vi "Create.vi"(8 "error in (no error)":errorcluster, 10 "Channel":T1=1 items=["ENC1"=1, "ENC2"=2], 11 "connection ID":i32=-1) -> (0 "error out":errorcluster, 3 "Task out":refnum<class "Encoder.lvclass">)   [LabVIEW 2009, in "MicroDAQ.lvlib" / "Encoder.lvclass"]
uses:
  <instrlib>/MicroDAQ/Channel/Encoder/Encoder.lvclass
  <instrlib>/MicroDAQ/Tools/Encoder type.ctl
  <instrlib>/MicroDAQ/Channel/Encoder/Encoder.lvclass/Encoder.ctl
  <instrlib>/MicroDAQ/Mlink library wraper/mlink.lvlib
  <instrlib>/MicroDAQ/Channel/Channel.lvclass
  <instrlib>/MicroDAQ/MicroDAQ.lvlib
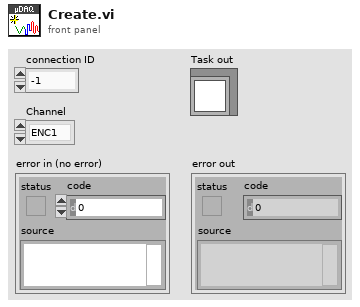
[diagram p1: front panel]
types:
  T1 = typedef "MicroDAQ.lvlib/Encoder type.ctl" = u8
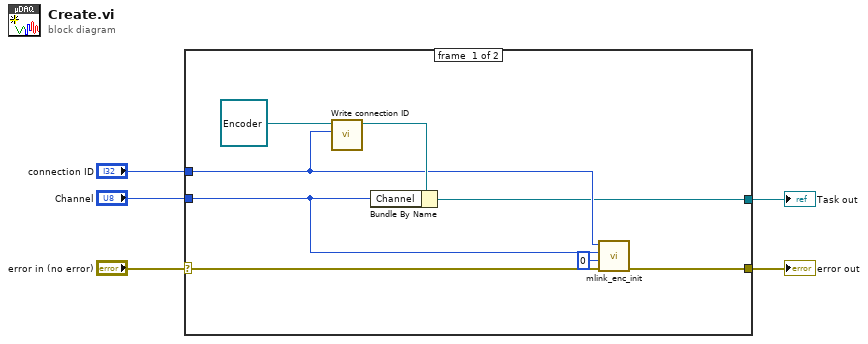
[diagram p0: block diagram]
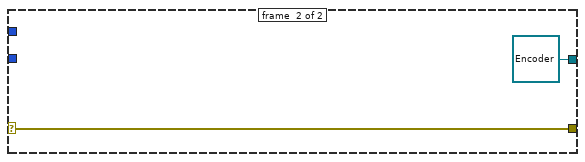
[diagram p2: hidden frame]
diagram:
  n1 = case shown="No Error" "error in (no error)" {
    selector: "error in (no error)" -> [w13 w15]
    tunnel: [w12 w15] -> w4
    tunnel: "Channel" -> [w8 _]
    tunnel: "connection ID" -> [w9 _]
    tunnel: [w6 refnum<class "Encoder.lvclass"> refnum ("Task out")] -> w1
    frame #0 {
      n2 = call <instrlib>:"Write connection ID.vi"("connection ID"=w9, "Task in"=refnum<class "Encoder.lvclass"> refnum ("MicroDAQ.lvlib:Encoder.lvclass 2")) -> ("Task out"=w10:refnum<class "Encoder.lvclass">)  [unwired: 9 in]
      n3 = Bundle By Name(cluster=w10, "Channel"=w8) -> (w6:refnum<class "Encoder.lvclass">)
      n4 = call <instrlib>:"mlink_enc_init.vi"("error in (no error)"=w13, "init value"=0, "channel"=w8, "connection ID"=w9) -> ("error out"=w12:errorcluster)  [unwired: 6 in, 1 out]
    }
    frame #1 {
    }
  }
  "error out" <- w4
  "Task out" <- w1
